vi "WFPropertiesAssemble.vi"(8 "Duration (s)":dbl=0.1 min=0.0, 9 "Ramp (s)":dbl=0.02 min=0.0, 10 "Amplitude (V)":dbl=5.0, 11 "Fs (Hz)":dbl=20000.0 min=0.0) -> (3 "Waveform Properties":T1={"Fs (Hz)"=20000.0, "Amplitude (V)"=5.0, "Ramp (s)"=0.02, "Duration (s)"=0.1} {"Ramp (s)" min=0.0; "Fs (Hz)" min=0.0})   [LabVIEW 2013]
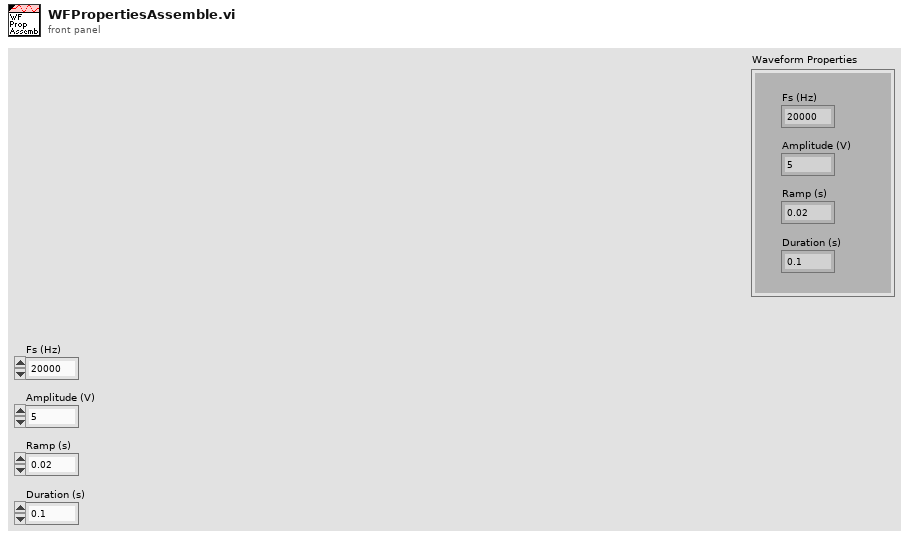
[diagram p1: front panel]
types:
  T1 = cluster{"Fs (Hz)":dbl, "Amplitude (V)":dbl, "Ramp (s)":dbl, "Duration (s)":dbl}
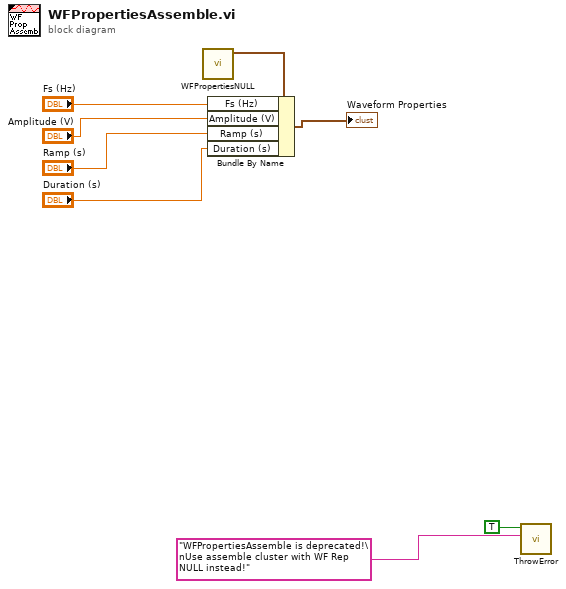
[diagram p0: block diagram]
diagram:
  n1 = call "WFPropertiesNULL.vi"() -> ("Waveform Properties"=w6:T1)  [unwired: 11 in]
  n2 = Bundle By Name(cluster=w6, "Fs (Hz)"="Fs (Hz)", "Amplitude (V)"="Amplitude (V)", "Ramp (s)"="Ramp (s)", "Duration (s)"="Duration (s)") -> (→"Waveform Properties":T1)
  n3 = call "ThrowError.vi"("Error Message"="WFPropertiesAssemble is deprecated!\nUse assemble cluster with WF Rep NULL instead!", "Error Input"=TRUE) -> ()  [unwired: 8 in, 2 out]
